vi "ATM.vi"() -> ()   [LabVIEW 2023]
doc: "This is the Main VI that performs the AMT operations."
uses:
  Controls/Left_Menu_Dispaly.ctl
  Controls/Right_Menu_Display.ctl
  Controls/Queue_Operation_Select.ctl
  Controls/ATM_Data.ctl
  Controls/Control_Reference.ctl
  Controls/State_Data.ctl
  Controls/Notifier_Operation_Select.ctl
  Controls/Timer_Operation_Select.ctl
  Controls/File_Operation_Select.ctl
panel:
  in  "User_Input":string caption="User Input"
  out "Error_Out":errorcluster
  in  "Error_In":errorcluster
  out "ATM_Message":string caption="ATM Message"
  out "Right_Menu":T1 caption="Right Menu"
  out "Left_Menu":T2 caption="Left Menu"
  in  "Right_Buttons":T3 caption="Right Buttons"
  in  "Left_Buttons":T4 caption="Left Buttons"
  in  "Enter":bool
  in  "Card_Simulator":bool caption="Card Simulator"
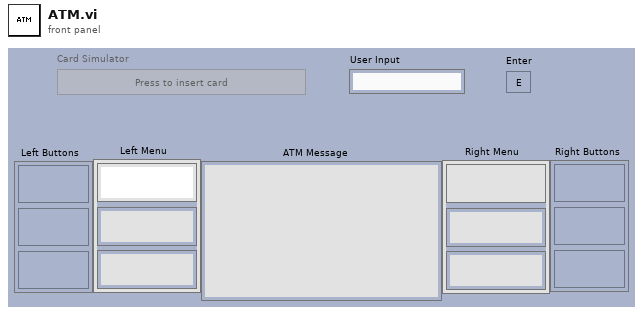
[diagram p1: front panel]
types:
  T1 = typedef "Right_Menu_Display.ctl" = cluster{"Withdraw_D":string, "Deposit_D":string, "Fast_cash_$50_D":string}
  T2 = typedef "Left_Menu_Dispaly.ctl" = cluster{"Balance_Inquiry_D":string, "None_D":string, "Return_Card_&_Terminate":string}
  T3 = cluster{"Deposit":bool, "Withdraw":bool, "Fast_Cash_$50":bool}
  T4 = cluster{"None":bool, "Balance_Inquiry":bool, "Return_Card_&_Terminate":bool}
  T5 = typedef "Notifier_Operation_Select.ctl" = enum16{"Obtain_Notification", "Send_Notification", "Get_Notification_Status", "Release_Notification"}
  T6 = typedef "Queue_Operation_Select.ctl" = enum16{"Obtain_Queue", "Enqueue", "Enqueue_N", "Enqueue_at_First", "Dequeue", "Flush_Queue", "Release_Queue"}
  T7 = typedef "Timer_Operation_Select.ctl" = enum16{"Start_Timer", "Time_Out?", "Stop_Timer"}
  T8 = typedef "State_Data.ctl" = cluster{"State":string, "Data":string}
  T9 = typedef "ATM_Data.ctl" = cluster{"Account_Details":string[][], "Selected_Account_Details":string[], "ATM_Message":string, "Left_Menu":T2, "Right_Menu":T1, "Contol_Buttons":refnum<vi>[], "Enter_&_User_Input":refnum<vi>[], "Card_Simulator":refnum<vi>[], "Disable_Control_Reference":refnum<vi>[], "Enable_Control_Reference":refnum<vi>[], "Control_Reference":T10, "Current_Process":string, "Event_Data":string, "Current_Banking_Process":string, "Selected_Banking":string, "Index_of_Selected_Account":i32, "Terminated?":bool}
  T10 = typedef "Control_Reference.ctl" = cluster{"User_Input":refnum<vi>, "Fast_Cash_$50":refnum<vi>, "Withdraw":refnum<vi>, "Deposit":refnum<vi>, "Return_Card_&_Terminate":refnum<vi>, "Balance_Inquiry":refnum<vi>, "None":refnum<vi>, "Enter":refnum<vi>, "Card_Simulator":refnum<vi>}
  T11 = typedef "File_Operation_Select.ctl" = enum16{"Get_Details", "Update_Details"}
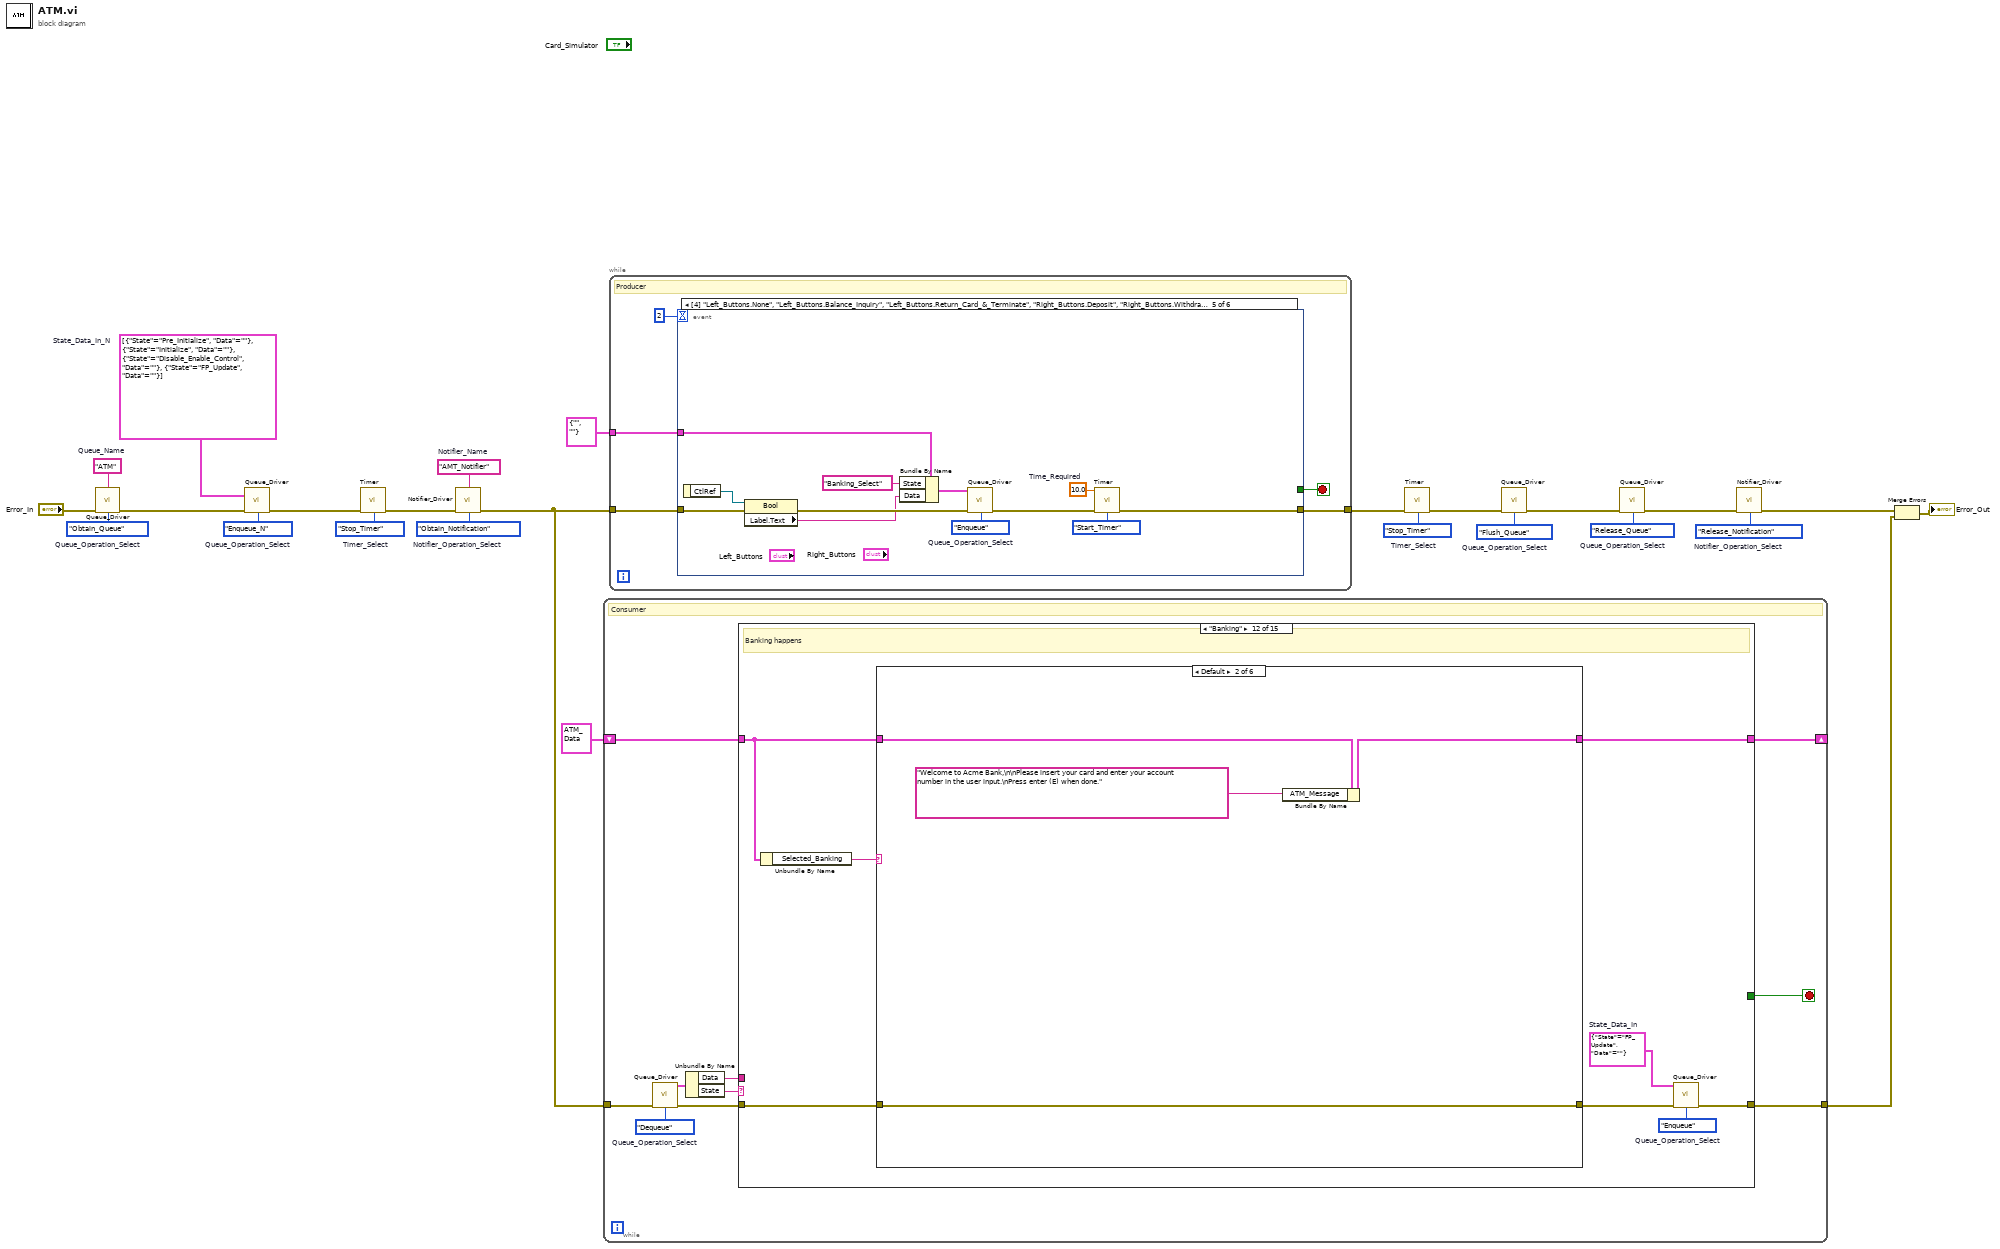
[diagram p0: block diagram]
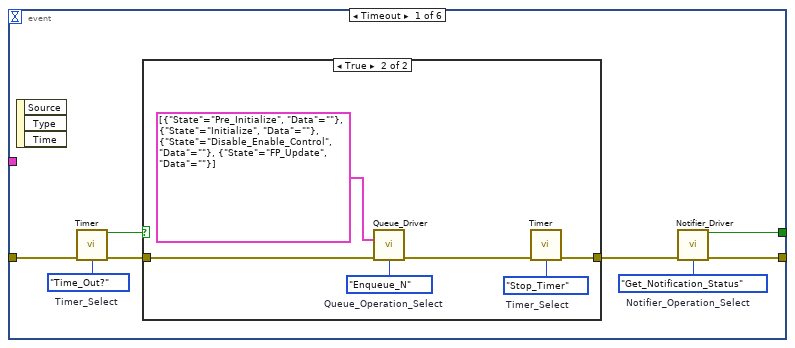
[diagram p2: hidden frame]
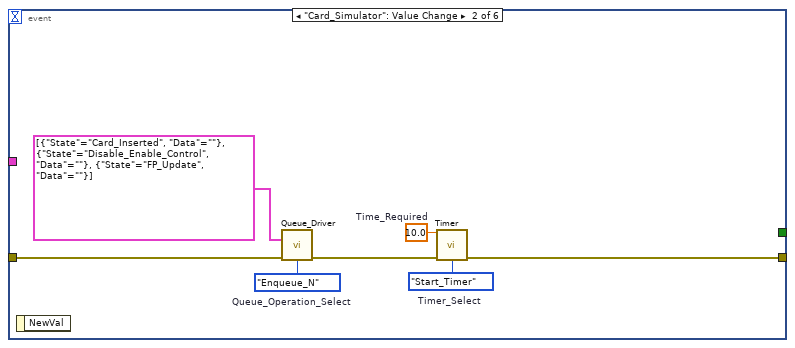
[diagram p4: hidden frame]
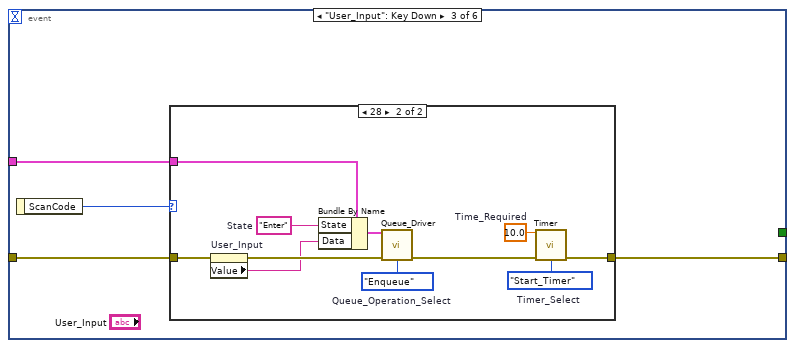
[diagram p5: hidden frame]
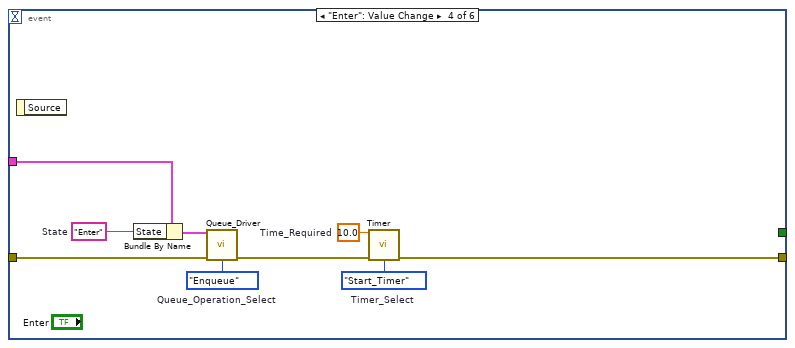
[diagram p7: hidden frame]
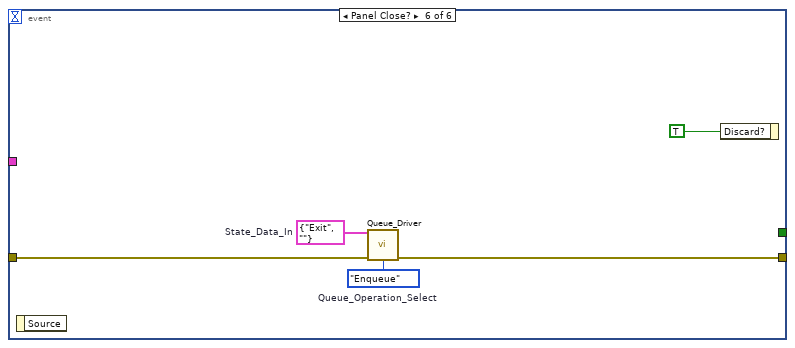
[diagram p8: hidden frame]
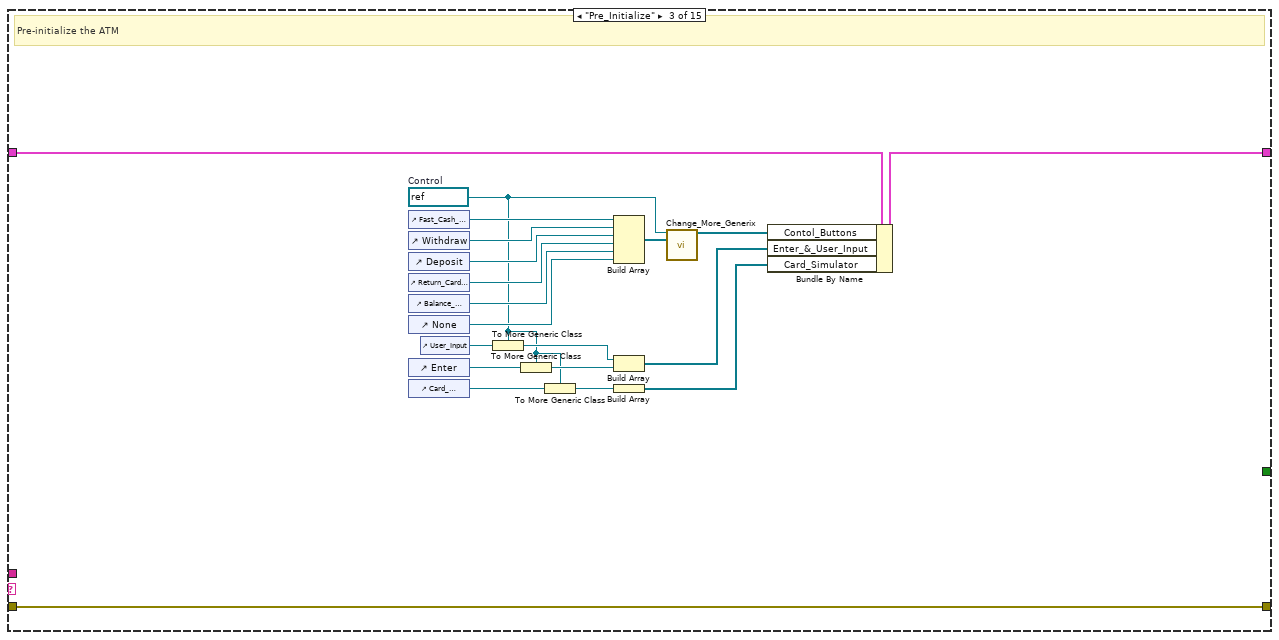
[diagram p11: hidden frame]
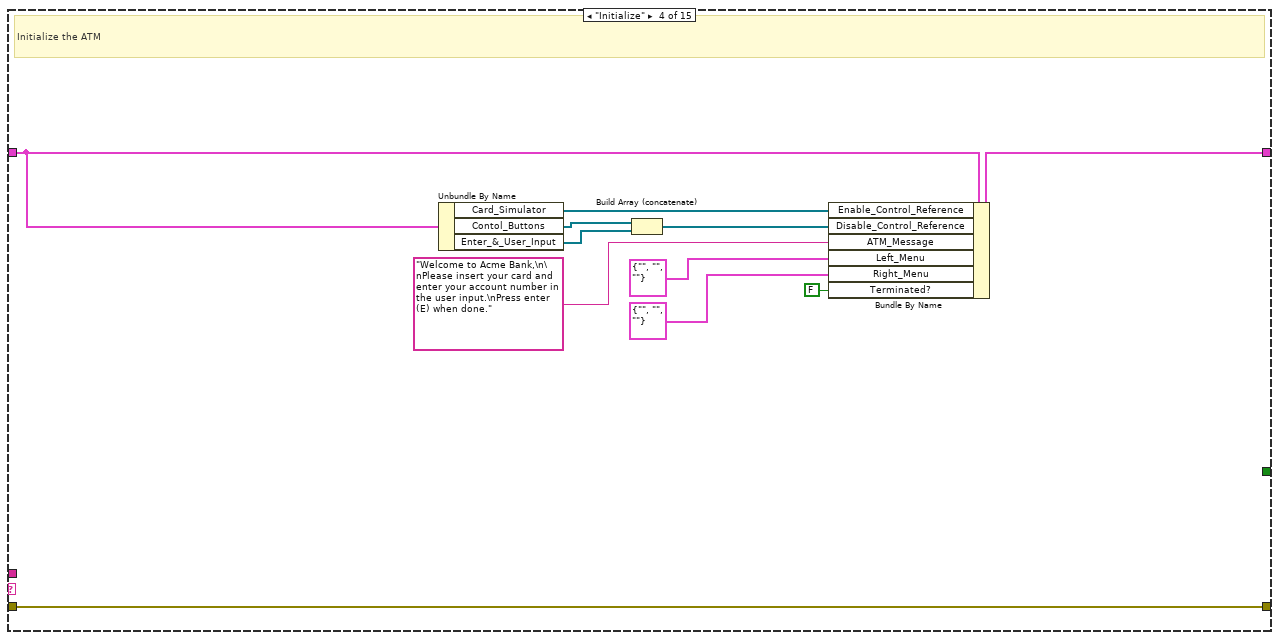
[diagram p12: hidden frame]
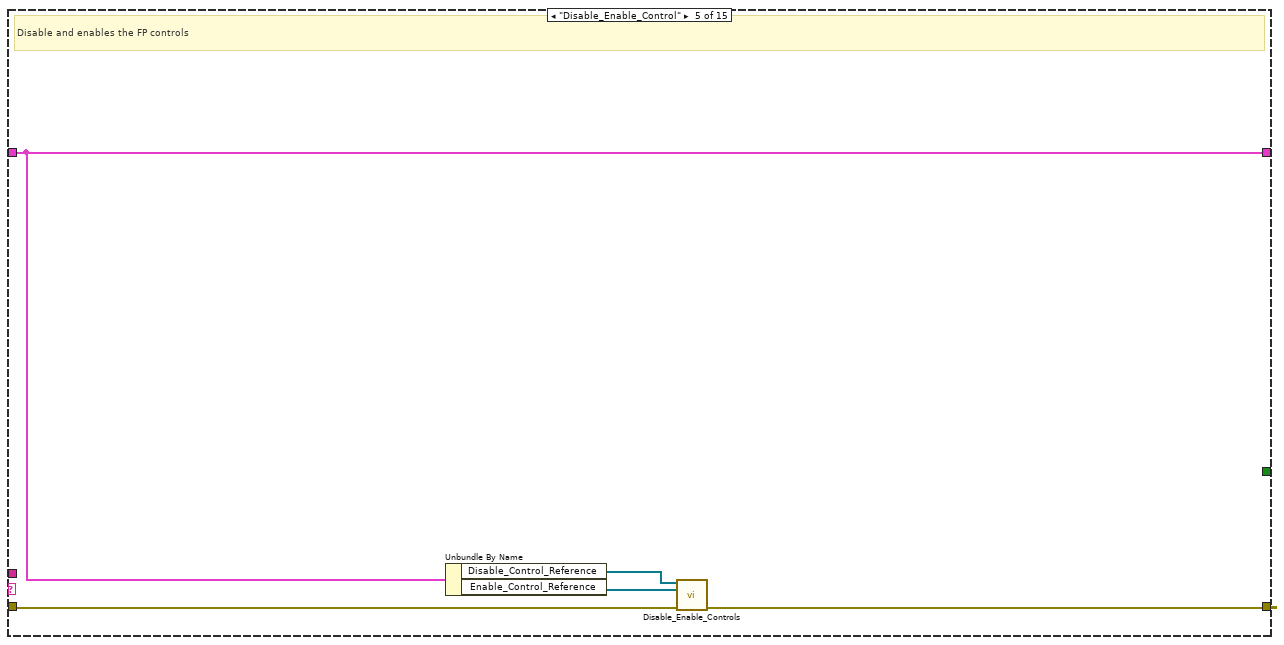
[diagram p13: hidden frame]
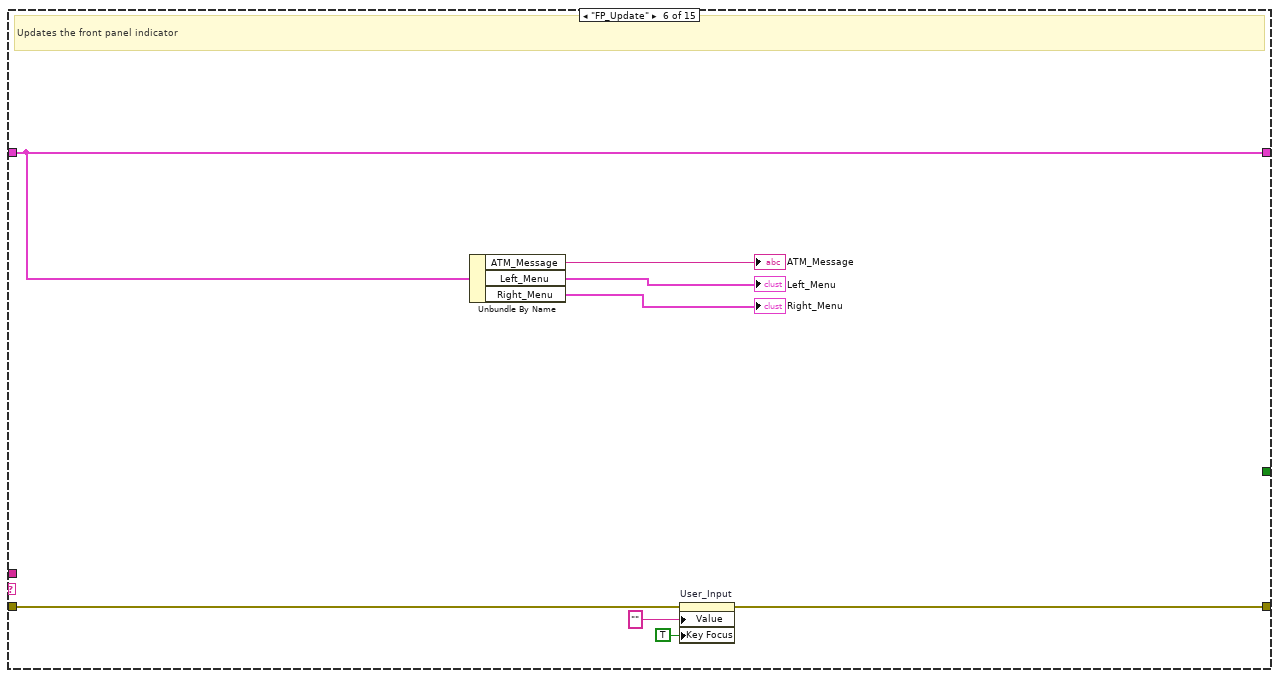
[diagram p14: hidden frame]
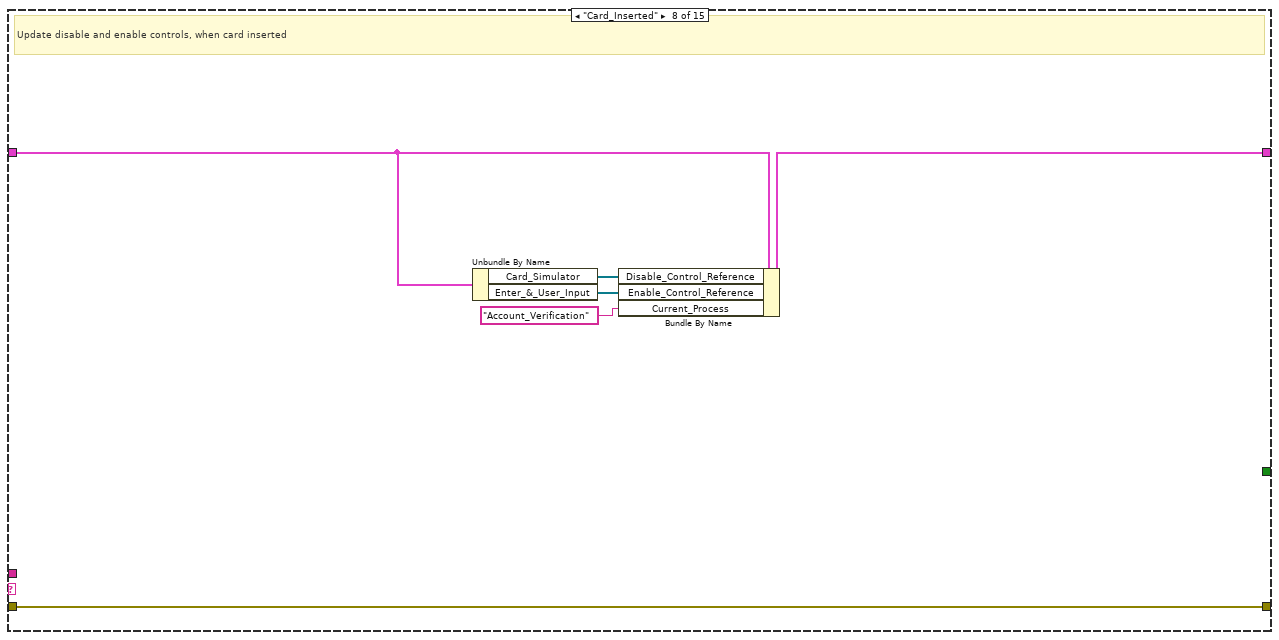
[diagram p16: hidden frame]
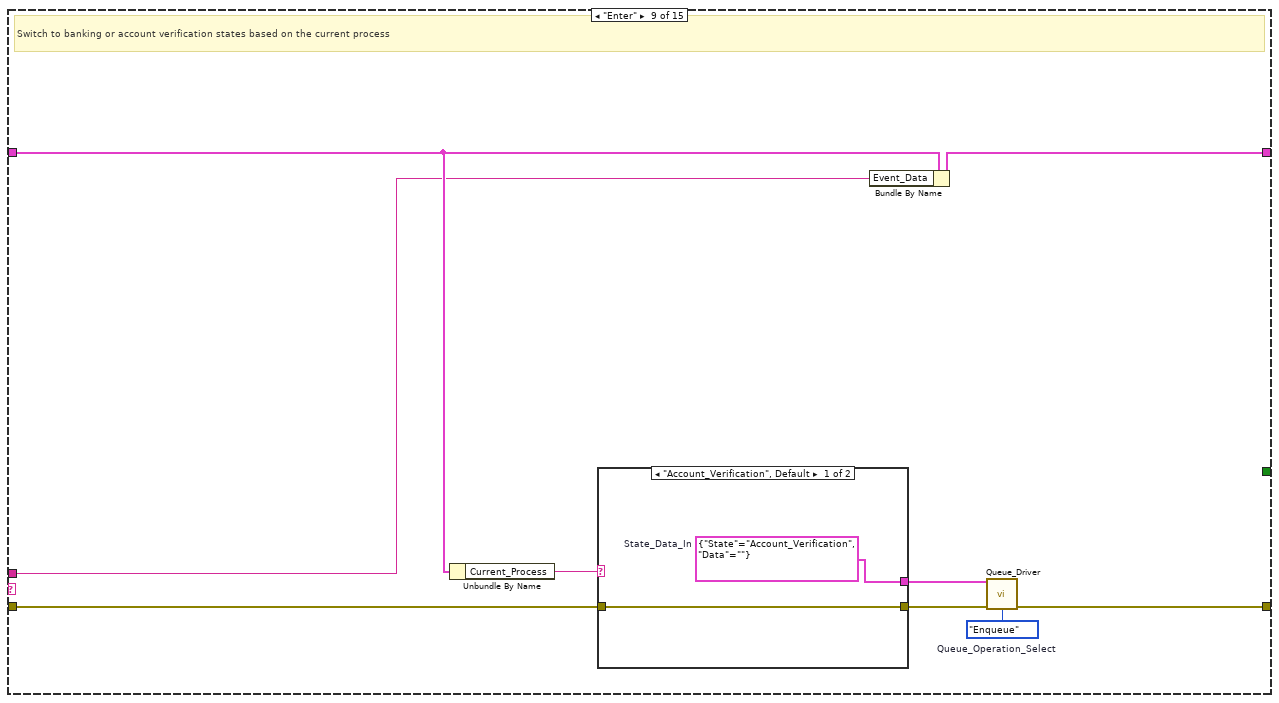
[diagram p17: hidden frame]
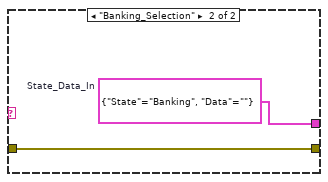
[diagram p18: hidden frame]
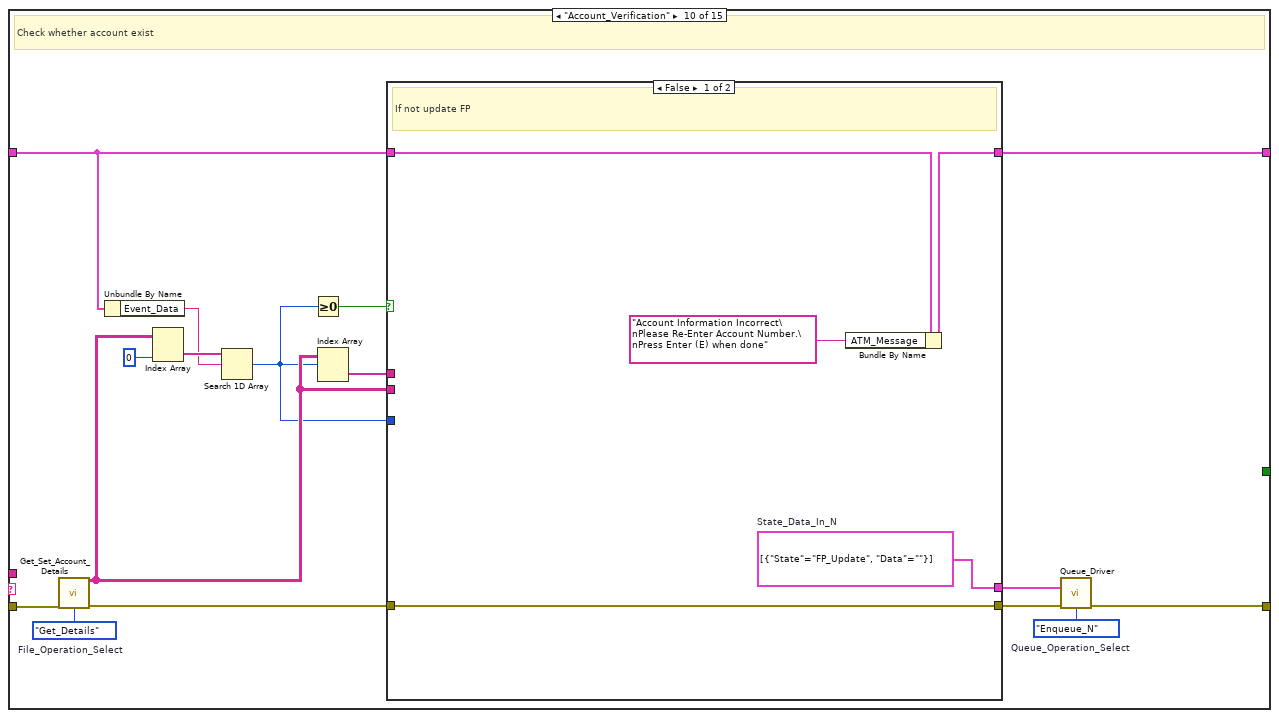
[diagram p19: hidden frame]
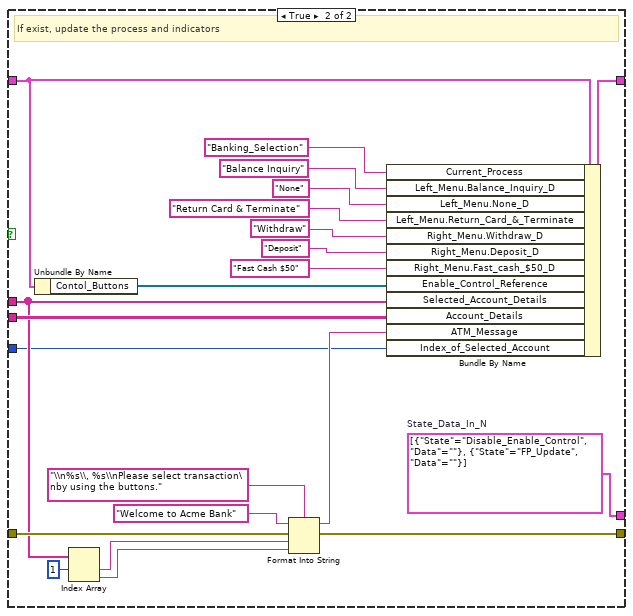
[diagram p20: hidden frame]
diagram:
  w1 = Notifier_Operation_Select."Release_Notification"  # Notifier_Operation_Select
  w2 = Queue_Operation_Select."Release_Queue"  # Queue_Operation_Select
  w4 = Queue_Operation_Select."Flush_Queue"  # Queue_Operation_Select
  w5 = Timer_Operation_Select."Stop_Timer"  # Timer_Select
  w9 = "AMT_Notifier"  # Notifier_Name
  w10 = Notifier_Operation_Select."Obtain_Notification"  # Notifier_Operation_Select
  w14 = Timer_Operation_Select."Stop_Timer"  # Timer_Select
  w17 = T8[] [{"State"="Pre_Initialize", "Data"=""}, {"State"="Initialize", "Data"=""}, {"State"="Disable_Enable_Control", "Data"=""}, {"State"="FP_Update", "Data"=""}]  # State_Data_In_N
  w18 = Queue_Operation_Select."Enqueue_N"  # Queue_Operation_Select
  w21 = "ATM"  # Queue_Name
  w22 = Queue_Operation_Select."Obtain_Queue"  # Queue_Operation_Select
  n1 = call "Queue_Driver.vi"("Queue_Name"=w21, "Error_In"="Error_In", "Queue_Operation_Select"=w22) -> ("Error_Out"=w23:errorcluster)  [unwired: 11 in, 1 out]
  n2 = call "Queue_Driver.vi"("State_Data_In_N"=w17, "Error_In"=w23, "Queue_Operation_Select"=w18) -> ("Error_Out"=w19:errorcluster)  [unwired: 11 in, 1 out]
  n3 = call "Timer.vi"("Error_In"=w19, "Timer_Select"=w14) -> ("Error_Out"=w15:errorcluster)  [unwired: 12 in, 1 out]
  n4 = call "Notifier_Driver.vi"("Notifier_Name"=w9, "Error_In"=w15, "Notifier_Operation_Select"=w10) -> ("Error_Out"=w11:errorcluster)  [unwired: 11 in, 1 out]
  n5 = while {
    tunnel: w11 -> [w35]
    tunnel: [w34] -> w12
    shift-right: [w28] -> _
    shift-left: T9 {"Account_Details"=[], "Selected_Account_Details"=[], "ATM_Message"="", "Left_Menu"={"Balance_Inquiry_D"="", "None_D"="", "Return_Card_&_Terminate"=""}, "Right_Menu"={"Withdraw_D"="", "Deposit_D"="", "Fast_cash_$50_D"=""}, "Contol_Buttons"=[], "Enter_&_User_Input"=[], "Card_Simulator"=[], "Disable_Control_Reference"=[], "Enable_Control_Reference"=[], "Control_Reference"={"User_Input"=refnum, "Fast_Cash_$50"=refnum, "Withdraw"=refnum, "Deposit"=refnum, "Return_Card_&_Terminate"=refnum, "Balance_Inquiry"=refnum, "None"=refnum, "Enter"=refnum, "Card_Simulator"=refnum}, "Current_Process"="", "Event_Data"="", "Current_Banking_Process"="", "Selected_Banking"="", "Index_of_Selected_Account"=0, "Terminated?"=FALSE} -> [w29]
    stop <- w26 stop-if-true
    w32 = Queue_Operation_Select."Dequeue"  # Queue_Operation_Select
    # "Consumer"
    n6 = call "Queue_Driver.vi"("Error_In"=w35, "Queue_Operation_Select"=w32) -> ("State_Data_Out"=w30:T8, "Error_Out"=w33:errorcluster)  [unwired: 12 in]
    n7 = Unbundle By Name(w30) -> ("Data"=w27:string, "State"=w31:string)
    n8 = case shown="\"Banking\"" w31 {
      tunnel: w33 -> [w37 w39 w59 w70 w75 w81 w85 w86 w99 w120 w162 w200 w292 w299 w313]
      tunnel: [w37 w39 w59 w70 w74 w80 w85 w86 w94 w108 w155 w195 w292 w298 w315] -> w34
      tunnel: w29 -> [w36 w38 w58 w69 w71 w83 w84 w90 w97 w118 w148 w198 w291 w310 w316]
      tunnel: [w36 w38 w57 w68 w71 w83 w84 w91 w96 w114 w161 w201 w291 w310 w316] -> w28
      tunnel: w27 -> [_ _ _ _ _ _ _ _ w95 _ w159 _ _ _ _]
      tunnel: [_ _ _ _ _ _ _ _ _ _ _ _ _ _ w311] -> w26
      frame Default {
        # "Default"
      }
      frame "---Initialize_and_Update_Front_Panel---" {
        # "States after this are initialization and front panel updation"
      }
      frame "Pre_Initialize" {
        w42 = refnum<vi> refnum  # Control
        # "Pre-initialize the ATM"
        n9 = control-ref of="Fast_Cash_$50"() -> (w56:refnum<vi>)
        n10 = control-ref of="Withdraw"() -> (w55:refnum<vi>)
        n11 = control-ref of="Deposit"() -> (w54:refnum<vi>)
        n12 = control-ref of="Return_Card_&_Terminate"() -> (w53:refnum<vi>)
        n13 = control-ref of="Balance_Inquiry"() -> (w52:refnum<vi>)
        n14 = control-ref of="None"() -> (w47:refnum<vi>)
        n15 = control-ref of="Enter"() -> (w49:refnum<vi>)
        n16 = control-ref of="Card_Simulator"() -> (w41:refnum<vi>)
        n17 = control-ref of="User_Input"() -> (w40:refnum<vi>)
        n18 = To More Generic Class(target class=w42, reference=w40) -> (generic class reference=w48:refnum<vi>)
        n19 = To More Generic Class(target class=w42, reference=w49) -> (generic class reference=w45:refnum<vi>)
        n20 = To More Generic Class(target class=w42, reference=w41) -> (generic class reference=w43:refnum<vi>)
        n21 = Build Array(w56, w55, w54, w53, w52, w47) -> (w51:refnum<vi>[])
        n22 = Build Array(w48, w45) -> (w46:refnum<vi>[])
        n23 = Build Array(w43) -> (w44:refnum<vi>[])
        n24 = call "Change_More_Generix.vi"("Control_In"=w42, "Reference_In"=w51) -> ("Reference_Out"=w50:refnum<vi>[])  [unwired: 13 in]
        n25 = Bundle By Name(cluster=w58, "Contol_Buttons"=w50, "Enter_&_User_Input"=w46, "Card_Simulator"=w44) -> (w57:T9)
      }
      frame "Initialize" {
        # "Initialize the ATM"
        n26 = Unbundle By Name(w69) -> ("Card_Simulator"=w63:refnum<vi>[], "Contol_Buttons"=w67:refnum<vi>[], "Enter_&_User_Input"=w66:refnum<vi>[])
        n27 = Build Array (concatenate)(w67, w66) -> (w65:refnum<vi>[])
        n28 = Bundle By Name(cluster=w69, "Enable_Control_Reference"=w63, "Disable_Control_Reference"=w65, "ATM_Message"="Welcome to Acme Bank,\n\nPlease insert your card and enter your account number in the user input.\nPress enter (E) when done.", "Left_Menu"=T2 {"Balance_Inquiry_D"="", "None_D"="", "Return_Card_&_Terminate"=""}, "Right_Menu"=T1 {"Withdraw_D"="", "Deposit_D"="", "Fast_cash_$50_D"=""}, "Terminated?"=FALSE) -> (w68:T9)
      }
      frame "Disable_Enable_Control" {
        # "Disable and enables the FP controls"
        n29 = Unbundle By Name(w71) -> ("Disable_Control_Reference"=w73:refnum<vi>[], "Enable_Control_Reference"=w72:refnum<vi>[])
        n30 = call "Disable_Enable_Controls.vi"("Disable_Control"=w73, "Enable_Control"=w72, "Error_In"=w75) -> ("Error_Out"=w74:errorcluster)  [unwired: 12 in]
      }
      frame "FP_Update" {
        # "Updates the front panel indicator"
        n31 = Unbundle By Name(w83) -> ("ATM_Message"=→"ATM_Message":string, "Left_Menu"=→"Left_Menu":T2, "Right_Menu"=→"Right_Menu":T1)
        n32 = property on="User_Input" class="Str"(error in=w81, "Value"="" ("User_Input"), "Key Focus"=TRUE) -> (error out=w80:errorcluster)  [unwired: 1 in, 1 out]
      }
      frame "-------------Banking_States-------------" {
        # "States after this are Banking stats"
      }
      frame "Card_Inserted" {
        # "Update disable and enable controls, when card inserted"
        n33 = Unbundle By Name(w90) -> ("Card_Simulator"=w88:refnum<vi>[], "Enter_&_User_Input"=w89:refnum<vi>[])
        n34 = Bundle By Name(cluster=w90, "Disable_Control_Reference"=w88, "Enable_Control_Reference"=w89, "Current_Process"="Account_Verification") -> (w91:T9)
      }
      frame "Enter" {
        w93 = Queue_Operation_Select."Enqueue"  # Queue_Operation_Select
        # "Switch to banking or account verification states based on the current process"
        n35 = Unbundle By Name(w97) -> ("Current_Process"=w100:string)
        n36 = case shown="\"Account_Verification\", Default" w100 {
          tunnel: w99 -> [w102 w104]
          tunnel: [w102 w104] -> w98
          tunnel: [w101 w103] -> w92
          frame "Account_Verification", Default {
            w101 = T8 {"State"="Account_Verification", "Data"=""}  # State_Data_In
          }
          frame "Banking_Selection" {
            w103 = T8 {"State"="Banking", "Data"=""}  # State_Data_In
          }
        }
        n37 = Bundle By Name(cluster=w97, "Event_Data"=w95) -> (w96:T9)
        n38 = call "Queue_Driver.vi"("State_Data_In"=w92, "Error_In"=w98, "Queue_Operation_Select"=w93) -> ("Error_Out"=w94:errorcluster)  [unwired: 11 in, 1 out]
      }
      frame "Account_Verification" {
        w107 = Queue_Operation_Select."Enqueue_N"  # Queue_Operation_Select
        w119 = File_Operation_Select."Get_Details"  # File_Operation_Select
        # "Check whether account exist"
        n39 = call "Get_Set_Account_Details.vi"("error in (no error)"=w120, "File_Operation_Select"=w119) -> ("Account_Details"=w113:string[][], "error out"=w111:errorcluster)  [unwired: 12 in]
        n40 = Unbundle By Name(w118) -> ("Event_Data"=w115:string)
        n41 = Index Array(array=w113, index (col)=0 ("disabled index (col)")) -> (element=w116:string[])  [unwired: 1 in]
        n42 = Search 1D Array(1D array=w116, element=w115) -> (index of element=w105:i32)  [unwired: 1 in]
        n43 = Greater Or Equal To 0?(x=w105) -> (x >= 0?=w110:bool)
        n44 = Index Array(array=w113, index (row)=w105) -> (element=w112:string[])  [unwired: 1 in]
        n45 = case shown="False" w110 {
          tunnel: w118 -> [w124 w144]
          tunnel: [w123 w147] -> w114
          tunnel: w113 -> [_ w146]
          tunnel: w112 -> [_ w139]
          tunnel: w111 -> [w125 w145]
          tunnel: [w125 w142] -> w109
          tunnel: [w121 w134] -> w106
          tunnel: w105 -> [_ w126]
          frame False {
            w121 = T8[] [{"State"="FP_Update", "Data"=""}]  # State_Data_In_N
            # "If not update FP"
            n46 = Bundle By Name(cluster=w124, "ATM_Message"="Account Information Incorrect\nPlease Re-Enter Account Number.\nPress Enter (E) when done") -> (w123:T9)
          }
          frame True {
            w134 = T8[] [{"State"="Disable_Enable_Control", "Data"=""}, {"State"="FP_Update", "Data"=""}]  # State_Data_In_N
            # "If exist, update the process and indicators"
            n47 = Unbundle By Name(w144) -> ("Contol_Buttons"=w143:refnum<vi>[])
            n48 = Index Array(array=w139, index #1=1 ("index")) -> (element #1=w137:string, element #2=w135:string)  [unwired: 1 in]
            n49 = Format Into String(format string="\\n%s\\, %s\\nPlease select transaction\nby using the buttons.", initial string="Welcome to Acme Bank", error in=w145, w137, w135) -> (resulting string=w140:string, error out=w142:errorcluster)
            n50 = Bundle By Name(cluster=w144, "Current_Process"="Banking_Selection", "Left_Menu.Balance_Inquiry_D"="Balance Inquiry", "Left_Menu.None_D"="None", "Left_Menu.Return_Card_&_Terminate"="Return Card & Terminate", "Right_Menu.Withdraw_D"="Withdraw", "Right_Menu.Deposit_D"="Deposit", "Right_Menu.Fast_cash_$50_D"="Fast Cash $50", "Enable_Control_Reference"=w143, "Selected_Account_Details"=w139, "Account_Details"=w146, "ATM_Message"=w140, "Index_of_Selected_Account"=w126) -> (w147:T9)
          }
        }
        n51 = call "Queue_Driver.vi"("State_Data_In_N"=w106, "Error_In"=w109, "Queue_Operation_Select"=w107) -> ("Error_Out"=w108:errorcluster)  [unwired: 11 in, 1 out]
      }
      frame "Banking_Select" {
        w151 = ""  # Default
        w154 = Queue_Operation_Select."Enqueue_N"  # Queue_Operation_Select
        # "Updates the Banking Selected"
        n52 = Unbundle By Name(w148) -> ("Terminated?"=w152:bool)
        n53 = Select(t=w151, s=w152, f=w159) -> (s? t:f=w153:string)
        n54 = case shown="\"Fast_Cash_$50\"" w153 {
          selector: w153 -> [w165 w169 w173 w177 w181 w186 _]
          tunnel: w162 -> [w166 w170 w174 w178 w183 w188 w193]
          tunnel: [w166 w170 w174 w178 w183 w188 w193] -> w156
          tunnel: [_ _ _ _ "Please enter amount to deposit and press\nEnter (E) when done" "Please enter amount to withdraw and press\nEnter (E) when done" _] -> w160
          tunnel: [_ _ _ _ _ _ "50" ("Event_Data")] -> w158
          tunnel: [w165 w169 w173 w177 w181 w186 "Withdraw"] -> w157
          tunnel: [w164 w168 w172 w175 w180 w185 w190] -> w150
          tunnel: [w163 w167 w171 w176 w179 w184 w189] -> w149
          tunnel: w148 -> [w163 w167 w171 w176 w179 w184 w189]
          frame Default {
            w164 = T8[] [{"State"="Pre_Initialize", "Data"=""}, {"State"="Initialize", "Data"=""}, {"State"="Disable_Enable_Control", "Data"=""}, {"State"="FP_Update", "Data"=""}]  # State_Data_In_N
            # "Re initialize, if terminated and button pressed"
          }
          frame "Return_Card_&_Terminate" {
            w168 = T8[] [{"State"="Banking", "Data"=""}]  # State_Data_In
            # "Terminate the session"
          }
          frame "Balance_Inquiry" {
            w172 = T8[] [{"State"="Banking", "Data"=""}]  # State_Data_In
            # "Switch to Banking and get the balance"
          }
          frame "None" {
            w175 = T8[] []  # State_Data_In
            # "#Future updates"
          }
          frame "Deposit" {
            w180 = T8[] [{"State"="FP_Update", "Data"=""}]  # State_Data_In
            # "Update FP and with for Amount enter"
          }
          frame "Withdraw" {
            w185 = T8[] [{"State"="FP_Update", "Data"=""}]  # State_Data_In
            # "Update FP and wait for withdraw amount"
          }
          frame "Fast_Cash_$50" {
            w190 = T8[] [{"State"="Banking", "Data"=""}]  # State_Data_In
            # "Switch to banking and debit 50"
          }
        }
        n55 = Bundle By Name(cluster=w149, "ATM_Message"=w160, "Event_Data"=w158, "Selected_Banking"=w157) -> (w161:T9)
        n56 = call "Queue_Driver.vi"("State_Data_In_N"=w150, "Error_In"=w156, "Queue_Operation_Select"=w154) -> ("Error_Out"=w155:errorcluster)  [unwired: 11 in, 1 out]
      }
      frame "Banking" {
        w196 = T8 {"State"="FP_Update", "Data"=""}  # State_Data_In
        w197 = Queue_Operation_Select."Enqueue"  # Queue_Operation_Select
        # "Banking happens"
        n57 = Unbundle By Name(w198) -> ("Selected_Banking"=w194:string)
        n58 = case shown="Default" w194 {
          tunnel: w198 -> [w213 w219 w226 w229 w231 w270]
          tunnel: [w215 w217 w221 w229 w232 w271] -> w201
          tunnel: w200 -> [w211 w218 w227 w228 w233 w272]
          tunnel: [w206 w218 w227 w228 w234 w264] -> w199
          frame "Return_Card_&_Terminate" {
            w204 = 3.0  # Time_Required
            w205 = Timer_Operation_Select."Start_Timer"  # Timer_Select
            w212 = File_Operation_Select."Update_Details"  # File_Operation_Select
            # "Terminate the session"
            n59 = Unbundle By Name(w213) -> ("Account_Details"=w210:string[][], "Index_of_Selected_Account"=w209:i32, "Selected_Account_Details"=w208:string[])
            n60 = Replace Array Subset(array=w210, new element=w208, index (row)=w209) -> (w207:string[][])  [unwired: 1 in]
            n61 = call "Get_Set_Account_Details.vi"("Updated_Account_Details"=w207, "error in (no error)"=w211, "File_Operation_Select"=w212) -> ("error out"=w203:errorcluster)  [unwired: 11 in, 1 out]
            n62 = Bundle By Name(cluster=w213, "ATM_Message"="Your session has been terminated\ndue to inactivity or menu selection,\nPlease take your card\nGoodbye!", "Terminated?"=TRUE) -> (w215:T9)
            n63 = call "Timer.vi"("Time_Required"=w204, "Error_In"=w203, "Timer_Select"=w205) -> ("Error_Out"=w206:errorcluster)  [unwired: 11 in, 1 out]
          }
          frame Default {
            n64 = Bundle By Name(cluster=w219, "ATM_Message"="Welcome to Acme Bank,\n\nPlease insert your card and enter your account number in the user input.\nPress enter (E) when done.") -> (w217:T9)
          }
          frame "Balance_Inquiry" {
            w222 = "Your Balance Is:\n$ "  # Message
            w224 = 3  # Balance_Index
            # "Get the balance from the account"
            n65 = Unbundle By Name(w226) -> ("Selected_Account_Details"=w225:string[])
            n66 = Index Array(array=w225, index=w224) -> (element=w223:string)
            n67 = Concatenate Strings(w222, w223) -> (w220:string)
            n68 = Bundle By Name(cluster=w226, "ATM_Message"=w220) -> (w221:T9)
          }
          frame "None" {
            # "#FutureUpdate"
          }
          frame "Withdraw" {
            w240 = 3  # Balance_Index
            # "Withdraw the Amount from account"
            n69 = Unbundle By Name(w231) -> ("Selected_Account_Details"=w238:string[], "Event_Data"=w230:string)
            n70 = Index Array(array=w238, index=w240) -> (element=w239:string)
            n71 = Fract/Exp String To Number(string=w239) -> (number=w236:dbl)  [unwired: 3 in, 1 out]
            n72 = Fract/Exp String To Number(string=w230) -> (number=w235:dbl)  [unwired: 3 in, 1 out]
            n73 = Greater Or Equal?(x=w236, y=w235) -> (x >= y?=w237:bool)
            n74 = case shown="True" w237 {
              tunnel: w238 -> [_ w260]
              tunnel: w236 -> [_ w259]
              tunnel: w235 -> [_ w258]
              tunnel: [w244 w250] -> w234
              tunnel: w233 -> [w244 w254]
              tunnel: [w242 w252] -> w232
              tunnel: w231 -> [w243 w253]
              tunnel: w230 -> [_ w247]
              frame False {
                # "If Insufficient"
                n75 = Bundle By Name(cluster=w243, "ATM_Message"="Insufficient funds in account\nPlease check your balance\nand try again") -> (w242:T9)
              }
              frame True {
                w248 = "%s Withdrawn"  # Format
                w249 = "$ "  # Dollar
                w255 = 3  # Balance_Index
                # "If Sufficient"
                n76 = Subtract(x=w259, y=w258) -> (x-y=w257:dbl)
                n77 = Number To Fractional String(number=w257) -> (F-format string=w256:string)  [unwired: 3 in]
                n78 = Replace Array Subset(array=w260, new element=w256, index=w255) -> (w251:string[])
                n79 = Format Into String(format string=w248, initial string=w249, error in=w254, w247) -> (resulting string=w246:string, error out=w250:errorcluster)
                n80 = Bundle By Name(cluster=w253, "Selected_Account_Details"=w251, "ATM_Message"=w246, "Selected_Banking"="") -> (w252:T9)
              }
            }
          }
          frame "Deposit" {
            w265 = 3  # Balance_Index
            # "Deposit the Amount to the account"
            n81 = Unbundle By Name(w270) -> ("Selected_Account_Details"=w266:string[], "Event_Data"=w263:string)
            n82 = Fract/Exp String To Number(string=w263) -> (number=w262:dbl)  [unwired: 3 in, 1 out]
            n83 = Index Array(array=w266, index=w265) -> (element=w269:string)
            n84 = Fract/Exp String To Number(string=w269) -> (number=w268:dbl)  [unwired: 3 in, 1 out]
            n85 = Less Or Equal To 0?(x=w262) -> (x <= 0?=w261:bool)
            n86 = Add(x=w268, y=w262) -> (x+y=w267:dbl)
            n87 = case shown="False" w261 {
              tunnel: w272 -> [w286 w287]
              tunnel: [w285 w289] -> w271
              tunnel: w270 -> [w284 w290]
              tunnel: w267 -> [w283 _]
              tunnel: w266 -> [w282 _]
              tunnel: w265 -> [w280 _]
              tunnel: [w278 w287] -> w264
              tunnel: w263 -> [w274 _]
              frame False {
                w276 = "%s Deposited"  # Format
                w277 = "$"  # Dollar
                # "If sufficient amount"
                n88 = Number To Fractional String(number=w283) -> (F-format string=w279:string)  [unwired: 3 in]
                n89 = Format Into String(format string=w276, initial string=w277, error in=w286, w274) -> (resulting string=w275:string, error out=w278:errorcluster)
                n90 = Replace Array Subset(array=w282, new element=w279, index=w280) -> (w281:string[])
                n91 = Bundle By Name(cluster=w284, "Selected_Account_Details"=w281, "ATM_Message"=w275, "Selected_Banking"="") -> (w285:T9)
              }
              frame True {
                # "If In-sufficient amount"
                n92 = Bundle By Name(cluster=w290, "ATM_Message"="Add Sufficient Amount") -> (w289:T9)
              }
            }
          }
        }
        n93 = call "Queue_Driver.vi"("State_Data_In"=w196, "Error_In"=w199, "Queue_Operation_Select"=w197) -> ("Error_Out"=w195:errorcluster)  [unwired: 11 in, 1 out]
      }
      frame "----------Exception_Handling-----------" {
      }
      frame "Error_State" {
        w296 = T8 {"State"="Exit", "Data"=""}  # State_Data_In
        w297 = Queue_Operation_Select."Enqueue"  # Queue_Operation_Select
        w305 = "%d%s%s"  # Format_String
        w306 = "Application Error"  # Initial_String
        w307 = "Stop"  # T_Button
        w308 = "Continue"  # F_Button
        # "Handles the Error"
        n94 = call <vilib>:"Clear Errors.vi"("error in (no error)"=w299) -> ("error out"=w303:errorcluster)  [unwired: 5 in, 1 out]
        n95 = Unbundle By Name(w299) -> ("code"=w302:i32, "source"=w301:string)
        n96 = Format Into String(format string=w305, initial string=w306, error in=w303, w302, "\n", w301) -> (resulting string=w309:string, error out=w300:errorcluster)
        n97 = Two Button Dialog(message=w309, 1:w308, 2:w307) -> (T button?=w293:bool)
        n98 = Select(t=w296, s=w293, f=T8 {"State"="FP_Update", "Data"=""}) -> (s? t:f=w295:T8)
        n99 = call "Queue_Driver.vi"("State_Data_In"=w295, "Error_In"=w300, "Queue_Operation_Select"=w297) -> ("Error_Out"=w298:errorcluster)  [unwired: 11 in, 1 out]
      }
      frame "Exit" {
        w314 = Notifier_Operation_Select."Send_Notification"  # Notifier_Operation_Select
        # "Close the applicatiom"
        n100 = disable-structure shown="Default" {
          disable-tunnel: [w318 TRUE ("T button?")] -> w311
          disable-tunnel: w313 -> [w317 w322]
          disable-tunnel: [w317 w322] -> w312
          frame condition #0 (active) {
            w319 = "No"  # Continue_Exe
            w320 = "Yes"  # Stop_Exe
            w321 = "Do you want to stop the execution"  # Message
            # "Developer mode"
            n101 = Two Button Dialog(message=w321, 1:w319, 2:w320) -> (T button?=w318:bool)
          }
          frame condition #1 {
            # "Real time engine mode or application mode"
          }
        }
        n102 = call "Notifier_Driver.vi"("Notification"=w311, "Error_In"=w312, "Notifier_Operation_Select"=w314) -> ("Error_Out"=w315:errorcluster)  [unwired: 11 in, 1 out]
      }
    }
  }
  n103 = while {
    tunnel: [w327] -> w24
    tunnel: w11 -> [w328]
    tunnel: T8 {"State"="", "Data"=""} ("State_Data_In") -> [w326]
    stop <- w324 stop-if-true
    # "Producer"
    n104 = event shown="[4] \"Left_Buttons.None\", \"Left_Buttons.Balance_Inquiry\", \"Left_Buttons.Return_Card_&_Terminate\", \"Right_Buttons.Deposit\", \"Right_Buttons.Withdraw\", \"Right_Buttons.Fast_Cash_$50\": Value Change" {
      selector: _ -> [_ _ _ _ _ _]
      dyn-events: _ -> [_ _ _ _ _ _]
      timeout: 2 -> [_ _ _ _ _ _]
      tunnel: w328 -> [w336 w350 w354 w375 w387 w392]
      tunnel: [w331 w344 w353 w373 w378 w390] -> w327
      tunnel: w326 -> [_ _ w352 w374 w382 _]
      tunnel: [w329 _ _ _ _ _] -> w324
      event Timeout {
        w330 = Notifier_Operation_Select."Get_Notification_Status"  # Notifier_Operation_Select
        w333 = Timer_Operation_Select."Time_Out?"  # Timer_Select
        n105 = event-data() -> ()  [unwired: 1 in, 3 out]
        n106 = call "Timer.vi"("Error_In"=w336, "Timer_Select"=w333) -> ("Time_Out?"=w334:bool, "Error_Out"=w335:errorcluster)  [unwired: 12 in]
        n107 = case shown="True" w334 {
          tunnel: w335 -> [w337 w343]
          tunnel: [w337 w339] -> w332
          frame False {
          }
          frame True {
            w338 = Timer_Operation_Select."Stop_Timer"  # Timer_Select
            w341 = Queue_Operation_Select."Enqueue_N"  # Queue_Operation_Select
            n108 = call "Queue_Driver.vi"("State_Data_In_N"=T8[] [{"State"="Pre_Initialize", "Data"=""}, {"State"="Initialize", "Data"=""}, {"State"="Disable_Enable_Control", "Data"=""}, {"State"="FP_Update", "Data"=""}], "Error_In"=w343, "Queue_Operation_Select"=w341) -> ("Error_Out"=w342:errorcluster)  [unwired: 11 in, 1 out]
            n109 = call "Timer.vi"("Error_In"=w342, "Timer_Select"=w338) -> ("Error_Out"=w339:errorcluster)  [unwired: 12 in, 1 out]
          }
        }
        n110 = call "Notifier_Driver.vi"("Error_In"=w332, "Notifier_Operation_Select"=w330) -> ("Latest_Notification"=w329:bool, "Error_Out"=w331:errorcluster)  [unwired: 12 in]
      }
      event "Card_Simulator": Value Change {
        w346 = 10.0  # Time_Required
        w347 = Timer_Operation_Select."Start_Timer"  # Timer_Select
        w348 = Queue_Operation_Select."Enqueue_N"  # Queue_Operation_Select
        n111 = event-data() -> ()  [unwired: 1 in, 1 out]
        n112 = call "Queue_Driver.vi"("State_Data_In_N"=T8[] [{"State"="Card_Inserted", "Data"=""}, {"State"="Disable_Enable_Control", "Data"=""}, {"State"="FP_Update", "Data"=""}], "Error_In"=w350, "Queue_Operation_Select"=w348) -> ("Error_Out"=w349:errorcluster)  [unwired: 11 in, 1 out]
        n113 = call "Timer.vi"("Time_Required"=w346, "Error_In"=w349, "Timer_Select"=w347) -> ("Error_Out"=w344:errorcluster)  [unwired: 11 in, 1 out]
      }
      event "User_Input": Key Down {
        n114 = event-data() -> ("ScanCode"=w351:i16)  [unwired: 1 in]
        n115 = case shown="28" w351 {
          tunnel: w354 -> [w355 w358]
          tunnel: w352 -> [_ w362]
          tunnel: [w355 w361] -> w353
          frame 0, Default {
          }
          frame 28 {
            w359 = 10.0  # Time_Required
            w360 = Timer_Operation_Select."Start_Timer"  # Timer_Select
            w365 = "Enter"  # State
            w366 = Queue_Operation_Select."Enqueue"  # Queue_Operation_Select
            n116 = property on="User_Input" class="Str"(error in=w358) -> (error out=w357:errorcluster, "Value"=w356:string)  [unwired: 1 in, 1 out]
            n117 = Bundle By Name(cluster=w362, "State"=w365, "Data"=w356) -> (w363:T8)
            n118 = call "Queue_Driver.vi"("State_Data_In"=w363, "Error_In"=w357, "Queue_Operation_Select"=w366) -> ("Error_Out"=w364:errorcluster)  [unwired: 11 in, 1 out]
            n119 = call "Timer.vi"("Time_Required"=w359, "Error_In"=w364, "Timer_Select"=w360) -> ("Error_Out"=w361:errorcluster)  [unwired: 11 in, 1 out]
          }
        }
      }
      event "Enter": Value Change {
        w367 = 10.0  # Time_Required
        w368 = Timer_Operation_Select."Start_Timer"  # Timer_Select
        w371 = "Enter"  # State
        w372 = Queue_Operation_Select."Enqueue"  # Queue_Operation_Select
        n120 = event-data() -> ()  [unwired: 1 in, 1 out]
        n121 = Bundle By Name(cluster=w374, "State"=w371) -> (w369:T8)
        n122 = call "Queue_Driver.vi"("State_Data_In"=w369, "Error_In"=w375, "Queue_Operation_Select"=w372) -> ("Error_Out"=w370:errorcluster)  [unwired: 11 in, 1 out]
        n123 = call "Timer.vi"("Time_Required"=w367, "Error_In"=w370, "Timer_Select"=w368) -> ("Error_Out"=w373:errorcluster)  [unwired: 11 in, 1 out]
      }
      event "Left_Buttons.None", "Left_Buttons.Balance_Inquiry", "Left_Buttons.Return_Card_&_Terminate", "Right_Buttons.Deposit", "Right_Buttons.Withdraw", "Right_Buttons.Fast_Cash_$50": Value Change {
        w376 = 10.0  # Time_Required
        w383 = Queue_Operation_Select."Enqueue"  # Queue_Operation_Select
        n124 = event-data() -> ("CtlRef"=w385:refnum<vi>)  [unwired: 1 in]
        n125 = property class="Bool"(reference=w385, error in=w387) -> (error out=w386:errorcluster, "Label.Text"=w380:string)  [unwired: 1 out]
        n126 = Bundle By Name(cluster=w382, "State"="Banking_Select", "Data"=w380) -> (w381:T8)
        n127 = call "Queue_Driver.vi"("State_Data_In"=w381, "Error_In"=w386, "Queue_Operation_Select"=w383) -> ("Error_Out"=w384:errorcluster)  [unwired: 11 in, 1 out]
        n128 = call "Timer.vi"("Time_Required"=w376, "Error_In"=w384, "Timer_Select"=Timer_Operation_Select."Start_Timer") -> ("Error_Out"=w378:errorcluster)  [unwired: 11 in, 1 out]
      }
      event Panel Close? {
        w388 = T8 {"State"="Exit", "Data"=""}  # State_Data_In
        w389 = Queue_Operation_Select."Enqueue"  # Queue_Operation_Select
        n129 = event-data() -> ()  [unwired: 1 in, 1 out]
        n130 = call "Queue_Driver.vi"("State_Data_In"=w388, "Error_In"=w392, "Queue_Operation_Select"=w389) -> ("Error_Out"=w390:errorcluster)  [unwired: 11 in, 1 out]
        n131 = event-data("Discard?"=TRUE) -> ()  [unwired: 1 in, 1 out]
      }
    }
  }
  n132 = call "Timer.vi"("Error_In"=w24, "Timer_Select"=w5) -> ("Error_Out"=w7:errorcluster)  [unwired: 12 in, 1 out]
  n133 = call "Queue_Driver.vi"("Error_In"=w7, "Queue_Operation_Select"=w4) -> ("Error_Out"=w8:errorcluster)  [unwired: 12 in, 1 out]
  n134 = call "Queue_Driver.vi"("Error_In"=w8, "Queue_Operation_Select"=w2) -> ("Error_Out"=w3:errorcluster)  [unwired: 12 in, 1 out]
  n135 = call "Notifier_Driver.vi"("Error_In"=w3, "Notifier_Operation_Select"=w1) -> ("Error_Out"=w6:errorcluster)  [unwired: 12 in, 1 out]
  n136 = Merge Errors(w6, w12) -> (→"Error_Out":errorcluster)
